vi "RemoveSpursFromSweep.vi"(11 "sweep":cluster{"frequency":dbl[], "amplitude":dbl[]}) -> (3 "sweep":cluster{"frequency":dbl[], "amplitude":dbl[]})   [LabVIEW 2017, in "EmsaAnalysis.lvlib"]
uses:
  <vilib>/addons/InsightCM/Devices/Shared/Emsa/EmsaAnalysis/EmsaAnalysis.lvlib
  <vilib>/Analysis/NI_AALBase.lvlib
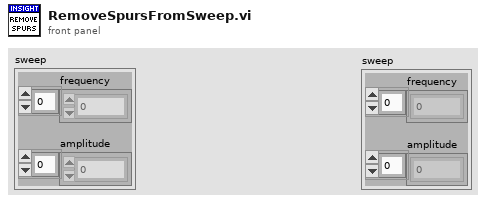
[diagram p1: front panel]
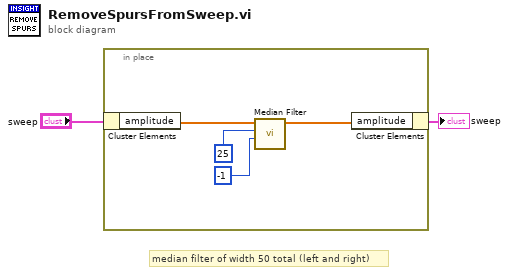
[diagram p0: block diagram]
diagram:
  # "median filter of width 50 total (left and right)"
  n1 = in-place {
    n2 = in-place-cluster #1("sweep") -> ("amplitude"=w4:dbl[])
    n3 = call <vilib>:"Median Filter.vi"("right rank"=-1, "left rank"=25, "X"=w4) -> ("Filtered X"=w3:dbl[])  [unwired: 7 in, 1 out]
    n4 = in-place-cluster #1("amplitude"=w3) -> (→"sweep":cluster{"frequency":dbl[], "amplitude":dbl[]})
  }
